vi "输入数据解析.vi"(0 "单个参数补充":dbl, 1 "从板号":dbl=1.0, 2 "主板二维码":string="BNET01", 3 "从板二维码":string="BNET01", 5 "主板引用":refnum<vi>, 7 "从板引用":refnum<vi>, 9 "主板选项":string="三级故障阀值", 11 "枚举":enum16{"主板", "从板"}(ring), 12 "快换":bool caption="快换写入") -> (4 "输出数组":dbl[][](array[numeric]), 6 "数组长度":dbl[](array[numeric]), 8 "循环次数":i32, 10 "命令":u32, 14 "名称":string[](array[string]), 15 "命令序号":u32[](array[numeric]))   [LabVIEW 2013] (continued)
                  disable-tunnel: [w3298 w3317] -> w3294
                  frame Disabled {
                    n1313 = Unbundle By Name(w3306) -> ("SOH过低"=w3305:dbl)
                    n1314 = call "输入分辨率计算-EV05.vi"("1字节?"=FALSE, "数值"=w3305, "偏移量"=0.0, "分辨率"=0.1) -> ("低字节"=w3307:dbl, "高字节1"=w3308:dbl)  [unwired: 1 in, 5 out]
                    n1315 = call "二进制解析-8.6.vi"("索引"=4, "数值"=w3308) -> ("低位子数组"=w3311:i32[])  [unwired: 3 out]
                    n1316 = call "二进制解析-8.6.vi"("索引"=4, "数值"=w3307) -> ("低位子数组"=w3300:i32[], "高位子数组"=w3310:i32[])  [unwired: 2 out]
                    n1317 = call "二进制解析-8.6.vi"("索引"=4, "数值"=0) -> ("低位子数组"=w3301:i32[])  [unwired: 3 out]
                    n1318 = Insert Into Array(array=w3311, new element=w3310) -> (w3304:i32[])  [unwired: 1 in]
                    n1319 = Insert Into Array(array=w3300, new element=w3301) -> (w3299:i32[])  [unwired: 1 in]
                    n1320 = call "数值二进制转十进制-8.6.vi"("子数组"=w3304) -> ("十进制数值"=w3309:i32)  [unwired: 4 out]
                    n1321 = call "数值二进制转十进制-8.6.vi"("子数组"=w3299) -> ("十进制数值"=w3298:i32)  [unwired: 4 out]
                  }
                  frame Enabled {
                    w3317 = 255 ("高字节1")
                  }
                }
                n1322 = Build Array(w3296, w3294) -> (w3297:i32[])
              }
            }
            n1323 = Insert Into Array(array=w3101, new element=w3102) -> (w3100:dbl[])  [unwired: 1 in]
          }
          n1324 = Build Array(w3097) -> (w3096:dbl[][])
          n1325 = Build Array("一级故障阀值") -> (w3087:string[])
        }
        frame "温度过低(2)" {
          n1326 = Unbundle By Name(w3323) -> ("一级故障 2"=w3324:refnum<vi>)
          n1327 = property class="Clust (严格)"(reference=w3324) -> ("Value"=w3322:T4)  [unwired: 1 in, 2 out]
          n1328 = for {
            N: 17 -> [_]
            tunnel: w3322 -> [w3334]
            shift-right: [w3331] -> w3328
            shift-left: dbl[] [] -> [w3332]
            i -> [w3335]
            n1329 = case shown="13" w3335 {
              tunnel: w3334 -> [w3336 w3347 w3358 w3368 w3378 w3388 w3400 w3412 w3424 w3436 w3448 w3460 w3474 w3496 w3508 w3517 w3526]
              tunnel: [w3337 w3348 w3359 w3369 w3379 w3390 w3402 w3414 w3426 w3438 w3450 w3461 w3483 w3499 w3507 w3516 w3528] -> w3333
              frame 0, Default {
                # "总电压过高"
                n1330 = disable-structure shown="启用" {
                  disable-tunnel: [w3343 w3346] -> w3339
                  disable-tunnel: [w3342 w3346] -> w3338
                  disable-tunnel: w3336 -> [w3341 _]
                  frame Disabled {
                    n1331 = Unbundle By Name(w3341) -> ("总电压过高"=w3340:dbl)
                    n1332 = call "输入分辨率计算-EV05.vi"("1字节?"=FALSE, "数值"=w3340, "分辨率"=0.1) -> ("低字节"=w3343:dbl, "高字节1"=w3342:dbl)  [unwired: 2 in, 5 out]
                  }
                  frame Enabled {
                    w3346 = 255 ("高字节1")
                  }
                }
                n1333 = Build Array(w3338, w3339) -> (w3337:i32[])
              }
              frame 1 {
                # "总电压过低"
                n1334 = disable-structure shown="启用" {
                  disable-tunnel: [w3354 w3357] -> w3350
                  disable-tunnel: [w3353 w3357] -> w3349
                  disable-tunnel: w3347 -> [w3352 _]
                  frame Disabled {
                    n1335 = Unbundle By Name(w3352) -> ("总电压过低"=w3351:dbl)
                    n1336 = call "输入分辨率计算-EV05.vi"("1字节?"=FALSE, "数值"=w3351, "分辨率"=0.1) -> ("低字节"=w3354:dbl, "高字节1"=w3353:dbl)  [unwired: 2 in, 5 out]
                  }
                  frame Enabled {
                    w3357 = 255 ("高字节1")
                  }
                }
                n1337 = Build Array(w3349, w3350) -> (w3348:i32[])
              }
              frame 2 {
                # "温度过高"
                n1338 = disable-structure shown="启用" {
                  disable-tunnel: [w3364 255 ("高字节1")] -> w3360
                  disable-tunnel: w3358 -> [w3362 _]
                  frame Disabled {
                    n1339 = Unbundle By Name(w3362) -> ("温度过高"=w3361:dbl)
                    n1340 = call "输入分辨率计算-EV05.vi"("1字节?"=TRUE, "数值"=w3361, "偏移量"=-40.0, "分辨率"=1.0) -> ("高字节1"=w3364:dbl)  [unwired: 1 in, 6 out]
                  }
                  frame Enabled {
                  }
                }
                n1341 = Build Array(w3360) -> (w3359:i32[])
              }
              frame 3 {
                # "温度过低"
                n1342 = disable-structure shown="启用" {
                  disable-tunnel: [w3374 255 ("高字节1")] -> w3370
                  disable-tunnel: w3368 -> [w3372 _]
                  frame Enabled {
                    n1343 = Unbundle By Name(w3372) -> ("温度过低"=w3371:dbl)
                    n1344 = call "输入分辨率计算-EV05.vi"("1字节?"=TRUE, "数值"=w3371, "偏移量"=-40.0, "分辨率"=1.0) -> ("高字节1"=w3374:dbl)  [unwired: 1 in, 6 out]
                  }
                  frame Disabled {
                  }
                }
                n1345 = Build Array(w3370) -> (w3369:dbl[])
              }
              frame 4 {
                # "整组温度不均衡"
                n1346 = disable-structure shown="启用" {
                  disable-tunnel: [w3384 255 ("高字节1")] -> w3380
                  disable-tunnel: w3378 -> [w3382 _]
                  frame Disabled {
                    n1347 = Unbundle By Name(w3382) -> ("整组温度不均衡"=w3381:dbl)
                    n1348 = call "输入分辨率计算-EV05.vi"("1字节?"=TRUE, "数值"=w3381, "偏移量"=0.0, "分辨率"=1.0) -> ("高字节1"=w3384:dbl)  [unwired: 1 in, 6 out]
                  }
                  frame Enabled {
                  }
                }
                n1349 = Build Array(w3380) -> (w3379:i32[])
              }
              frame 5 {
                # "单组电压不均衡"
                n1350 = disable-structure shown="启用" {
                  disable-tunnel: [w3396 w3399] -> w3391
                  disable-tunnel: [w3394 w3399] -> w3389
                  disable-tunnel: w3388 -> [w3393 _]
                  frame Disabled {
                    n1351 = Unbundle By Name(w3393) -> ("单组电压不均衡"=w3392:dbl)
                    n1352 = call "输入分辨率计算-EV05.vi"("1字节?"=FALSE, "数值"=w3392, "偏移量"=0.0, "分辨率"=0.001) -> ("低字节"=w3394:dbl, "高字节1"=w3396:dbl)  [unwired: 1 in, 5 out]
                  }
                  frame Enabled {
                    w3399 = 255 ("高字节1")
                  }
                }
                n1353 = Build Array(w3391, w3389) -> (w3390:i32[])
              }
              frame 6 {
                # "整组电压不均衡"
                n1354 = disable-structure shown="启用" {
                  disable-tunnel: [w3408 w3411] -> w3403
                  disable-tunnel: [w3406 w3411] -> w3401
                  disable-tunnel: w3400 -> [w3405 _]
                  frame Disabled {
                    n1355 = Unbundle By Name(w3405) -> ("整组电压不均衡"=w3404:dbl)
                    n1356 = call "输入分辨率计算-EV05.vi"("1字节?"=FALSE, "数值"=w3404, "偏移量"=0.0, "分辨率"=0.001) -> ("低字节"=w3406:dbl, "高字节1"=w3408:dbl)  [unwired: 1 in, 5 out]
                  }
                  frame Enabled {
                    w3411 = 255 ("高字节1")
                  }
                }
                n1357 = Build Array(w3403, w3401) -> (w3402:i32[])
              }
              frame 7 {
                # "单体电压过高"
                n1358 = disable-structure shown="启用" {
                  disable-tunnel: [w3420 w3423] -> w3415
                  disable-tunnel: [w3418 w3423] -> w3413
                  disable-tunnel: w3412 -> [w3417 _]
                  frame Disabled {
                    n1359 = Unbundle By Name(w3417) -> ("单体电压过高"=w3416:dbl)
                    n1360 = call "输入分辨率计算-EV05.vi"("1字节?"=FALSE, "数值"=w3416, "偏移量"=0.0, "分辨率"=0.001) -> ("低字节"=w3418:dbl, "高字节1"=w3420:dbl)  [unwired: 1 in, 5 out]
                  }
                  frame Enabled {
                    w3423 = 255 ("高字节1")
                  }
                }
                n1361 = Build Array(w3415, w3413) -> (w3414:i32[])
              }
              frame 8 {
                # "单体电压过低"
                n1362 = disable-structure shown="启用" {
                  disable-tunnel: [w3432 w3435] -> w3427
                  disable-tunnel: [w3430 w3435] -> w3425
                  disable-tunnel: w3424 -> [w3429 _]
                  frame Disabled {
                    n1363 = Unbundle By Name(w3429) -> ("单体电压过低"=w3428:dbl)
                    n1364 = call "输入分辨率计算-EV05.vi"("1字节?"=FALSE, "数值"=w3428, "偏移量"=0.0, "分辨率"=0.001) -> ("低字节"=w3430:dbl, "高字节1"=w3432:dbl)  [unwired: 1 in, 5 out]
                  }
                  frame Enabled {
                    w3435 = 255 ("高字节1")
                  }
                }
                n1365 = Build Array(w3427, w3425) -> (w3426:i32[])
              }
              frame 9 {
                # "充电电流过高"
                n1366 = disable-structure shown="启用" {
                  disable-tunnel: [w3444 w3447] -> w3439
                  disable-tunnel: [w3442 w3447] -> w3437
                  disable-tunnel: w3436 -> [w3441 _]
                  frame Disabled {
                    n1367 = Unbundle By Name(w3441) -> ("充电电流过高"=w3440:dbl)
                    n1368 = call "输入分辨率计算-EV05.vi"("1字节?"=FALSE, "数值"=w3440, "偏移量"=-3000.0, "分辨率"=0.1) -> ("低字节"=w3442:dbl, "高字节1"=w3444:dbl)  [unwired: 1 in, 5 out]
                  }
                  frame Enabled {
                    w3447 = 255 ("高字节1")
                  }
                }
                n1369 = Build Array(w3439, w3437) -> (w3438:i32[])
              }
              frame 10 {
                # "放电电流过高"
                n1370 = disable-structure shown="启用" {
                  disable-tunnel: [w3456 w3459] -> w3451
                  disable-tunnel: [w3454 w3459] -> w3449
                  disable-tunnel: w3448 -> [w3453 _]
                  frame Disabled {
                    n1371 = Unbundle By Name(w3453) -> ("放电电流过高"=w3452:dbl)
                    n1372 = call "输入分辨率计算-EV05.vi"("1字节?"=FALSE, "数值"=w3452, "偏移量"=-3000.0, "分辨率"=0.1) -> ("低字节"=w3454:dbl, "高字节1"=w3456:dbl)  [unwired: 1 in, 5 out]
                  }
                  frame Enabled {
                    w3459 = 255 ("高字节1")
                  }
                }
                n1373 = Build Array(w3451, w3449) -> (w3450:i32[])
              }
              frame 11 {
                # "单组温度不均衡"
                n1374 = disable-structure shown="启用" {
                  disable-tunnel: [w3466 255 ("高字节1")] -> w3462
                  disable-tunnel: w3460 -> [w3464 _]
                  frame Disabled {
                    n1375 = Unbundle By Name(w3464) -> ("单组温度不均衡"=w3463:dbl)
                    n1376 = call "输入分辨率计算-EV05.vi"("1字节?"=TRUE, "数值"=w3463, "偏移量"=0.0, "分辨率"=1.0) -> ("高字节1"=w3466:dbl)  [unwired: 1 in, 6 out]
                  }
                  frame Enabled {
                  }
                }
                n1377 = Build Array(w3462) -> (w3461:i32[])
              }
              frame 12 {
                # "SOC过高"
                n1378 = Unbundle By Name(w3474) -> ("SOC过高"=w3473:dbl)
                n1379 = call "输入分辨率计算-EV05.vi"("1字节?"=FALSE, "数值"=w3473, "偏移量"=0.0, "分辨率"=0.1) -> ("低字节"=w3475:dbl, "高字节1"=w3476:dbl)  [unwired: 1 in, 5 out]
                n1380 = call "二进制解析-8.6.vi"("索引"=4, "数值"=w3476) -> ("低位子数组"=w3479:i32[])  [unwired: 3 out]
                n1381 = call "二进制解析-8.6.vi"("索引"=4, "数值"=w3475) -> ("低位子数组"=w3471:i32[], "高位子数组"=w3478:i32[])  [unwired: 2 out]
                n1382 = Insert Into Array(array=w3479, new element=w3478) -> (w3477:i32[])  [unwired: 1 in]
                n1383 = call "数值二进制转十进制-8.6.vi"("子数组"=w3477) -> ("十进制数值"=w3472:i32)  [unwired: 4 out]
                n1384 = disable-structure shown="启用" {
                  disable-tunnel: w3472 -> [w3487 _]
                  disable-tunnel: [w3487 255 ("高字节1")] -> w3470
                  disable-tunnel: [w3486 i32[] [] ("低位子数组 21")] -> _
                  disable-tunnel: w3471 -> [w3486 _]
                  frame Disabled {
                  }
                  frame Enabled {
                  }
                }
                n1385 = Build Array(w3470, w3470) -> (w3483:i32[])
              }
              frame 13 {
                # "SOC过低"
                n1386 = Unbundle By Name(w3496) -> ("SOC过低"=w3495:dbl)
                n1387 = call "输入分辨率计算-EV05.vi"("1字节?"=FALSE, "数值"=w3495, "偏移量"=0.0, "分辨率"=0.1) -> ("低字节"=w3493:dbl, "高字节1"=w3494:dbl)  [unwired: 1 in, 5 out]
                n1388 = call "二进制解析-8.6.vi"("索引"=4, "数值"=w3494) -> ("低位子数组"=w3491:i32[])  [unwired: 3 out]
                n1389 = disable-structure shown="启用" {
                  disable-tunnel: w3493 -> [w3503 _]
                  disable-tunnel: [w3503 255 ("高字节1")] -> w3492
                  disable-tunnel: w3491 -> [w3502 _]
                  disable-tunnel: [_ 255 ("高字节1")] -> w3490
                  frame Disabled {
                    (unwired) i32[] [] ("低位子数组 4")
                  }
                  frame Enabled {
                  }
                }
                n1390 = Build Array(w3490, w3492) -> (w3499:i32[])
              }
              frame 14 {
                # "内阻过大"
                n1391 = disable-structure shown="启用" {
                  disable-tunnel: w3508 -> [w3513 _]
                  disable-tunnel: [w3509 255 ("高字节1")] -> w3506
                  frame Disabled {
                    n1392 = Unbundle By Name(w3513) -> ("内阻过大"=w3512:dbl)
                    n1393 = call "输入分辨率计算-EV05.vi"("1字节?"=TRUE, "数值"=w3512, "分辨率"=0.1) -> ("高字节1"=w3509:dbl)  [unwired: 2 in, 6 out]
                  }
                  frame Enabled {
                  }
                }
                n1394 = Build Array(w3506) -> (w3507:i32[])
              }
              frame 15 {
                # "极柱温度过高"
                n1395 = disable-structure shown="启用" {
                  disable-tunnel: w3517 -> [w3523 _]
                  disable-tunnel: [w3519 255 ("高字节1")] -> w3515
                  frame Disabled {
                    n1396 = Unbundle By Name(w3523) -> ("极柱温度过高"=w3522:dbl)
                    n1397 = call "输入分辨率计算-EV05.vi"("1字节?"=TRUE, "数值"=w3522, "偏移量"=-40.0, "分辨率"=1.0) -> ("高字节1"=w3519:dbl)  [unwired: 1 in, 6 out]
                  }
                  frame Enabled {
                  }
                }
                n1398 = Build Array(w3515) -> (w3516:i32[])
              }
              frame 16 {
                # "SOH过低"
                n1399 = disable-structure shown="启用" {
                  disable-tunnel: [w3540 w3548] -> w3527
                  disable-tunnel: w3526 -> [w3537 _]
                  disable-tunnel: [w3529 w3548] -> w3525
                  frame Disabled {
                    n1400 = Unbundle By Name(w3537) -> ("SOH过低"=w3536:dbl)
                    n1401 = call "输入分辨率计算-EV05.vi"("1字节?"=FALSE, "数值"=w3536, "偏移量"=0.0, "分辨率"=0.1) -> ("低字节"=w3538:dbl, "高字节1"=w3539:dbl)  [unwired: 1 in, 5 out]
                    n1402 = call "二进制解析-8.6.vi"("索引"=4, "数值"=w3539) -> ("低位子数组"=w3542:i32[])  [unwired: 3 out]
                    n1403 = call "二进制解析-8.6.vi"("索引"=4, "数值"=w3538) -> ("低位子数组"=w3531:i32[], "高位子数组"=w3541:i32[])  [unwired: 2 out]
                    n1404 = call "二进制解析-8.6.vi"("索引"=4, "数值"=0) -> ("低位子数组"=w3532:i32[])  [unwired: 3 out]
                    n1405 = Insert Into Array(array=w3542, new element=w3541) -> (w3535:i32[])  [unwired: 1 in]
                    n1406 = Insert Into Array(array=w3531, new element=w3532) -> (w3530:i32[])  [unwired: 1 in]
                    n1407 = call "数值二进制转十进制-8.6.vi"("子数组"=w3535) -> ("十进制数值"=w3540:i32)  [unwired: 4 out]
                    n1408 = call "数值二进制转十进制-8.6.vi"("子数组"=w3530) -> ("十进制数值"=w3529:i32)  [unwired: 4 out]
                  }
                  frame Enabled {
                    w3548 = 255 ("高字节1")
                  }
                }
                n1409 = Build Array(w3527, w3525) -> (w3528:i32[])
              }
            }
            n1410 = Insert Into Array(array=w3332, new element=w3333) -> (w3331:dbl[])  [unwired: 1 in]
          }
          n1411 = Build Array(w3328) -> (w3327:dbl[][])
          n1412 = Build Array("二级故障阀值") -> (w3318:string[])
        }
        frame "温度过低(3)" {
          n1413 = Unbundle By Name(w3554) -> ("一级故障 3"=w3555:refnum<vi>)
          n1414 = property class="Clust (严格)"(reference=w3555) -> ("Value"=w3553:T4)  [unwired: 1 in, 2 out]
          n1415 = for {
            N: 17 -> [_]
            tunnel: w3553 -> [w3565]
            shift-right: [w3562] -> w3559
            shift-left: dbl[] [] -> [w3563]
            i -> [w3566]
            n1416 = case shown="13" w3566 {
              tunnel: w3565 -> [w3567 w3578 w3589 w3599 w3609 w3619 w3631 w3643 w3655 w3667 w3679 w3691 w3705 w3727 w3739 w3748 w3757]
              tunnel: [w3568 w3579 w3590 w3600 w3610 w3621 w3633 w3645 w3657 w3669 w3681 w3692 w3714 w3730 w3738 w3747 w3759] -> w3564
              frame 0, Default {
                # "总电压过高"
                n1417 = disable-structure shown="启用" {
                  disable-tunnel: [w3574 w3577] -> w3570
                  disable-tunnel: [w3573 w3577] -> w3569
                  disable-tunnel: w3567 -> [w3572 _]
                  frame Disabled {
                    n1418 = Unbundle By Name(w3572) -> ("总电压过高"=w3571:dbl)
                    n1419 = call "输入分辨率计算-EV05.vi"("1字节?"=FALSE, "数值"=w3571, "分辨率"=0.1) -> ("低字节"=w3574:dbl, "高字节1"=w3573:dbl)  [unwired: 2 in, 5 out]
                  }
                  frame Enabled {
                    w3577 = 255 ("高字节1")
                  }
                }
                n1420 = Build Array(w3569, w3570) -> (w3568:i32[])
              }
              frame 1 {
                # "总电压过低"
                n1421 = disable-structure shown="启用" {
                  disable-tunnel: [w3585 w3588] -> w3581
                  disable-tunnel: [w3584 w3588] -> w3580
                  disable-tunnel: w3578 -> [w3583 _]
                  frame Disabled {
                    n1422 = Unbundle By Name(w3583) -> ("总电压过低"=w3582:dbl)
                    n1423 = call "输入分辨率计算-EV05.vi"("1字节?"=FALSE, "数值"=w3582, "分辨率"=0.1) -> ("低字节"=w3585:dbl, "高字节1"=w3584:dbl)  [unwired: 2 in, 5 out]
                  }
                  frame Enabled {
                    w3588 = 255 ("高字节1")
                  }
                }
                n1424 = Build Array(w3580, w3581) -> (w3579:i32[])
              }
              frame 2 {
                # "温度过高"
                n1425 = disable-structure shown="启用" {
                  disable-tunnel: [w3595 255 ("高字节1")] -> w3591
                  disable-tunnel: w3589 -> [w3593 _]
                  frame Disabled {
                    n1426 = Unbundle By Name(w3593) -> ("温度过高"=w3592:dbl)
                    n1427 = call "输入分辨率计算-EV05.vi"("1字节?"=TRUE, "数值"=w3592, "偏移量"=-40.0, "分辨率"=1.0) -> ("高字节1"=w3595:dbl)  [unwired: 1 in, 6 out]
                  }
                  frame Enabled {
                  }
                }
                n1428 = Build Array(w3591) -> (w3590:i32[])
              }
              frame 3 {
                # "温度过低"
                n1429 = disable-structure shown="启用" {
                  disable-tunnel: [w3605 255 ("高字节1")] -> w3601
                  disable-tunnel: w3599 -> [w3603 _]
                  frame Enabled {
                    n1430 = Unbundle By Name(w3603) -> ("温度过低"=w3602:dbl)
                    n1431 = call "输入分辨率计算-EV05.vi"("1字节?"=TRUE, "数值"=w3602, "偏移量"=-40.0, "分辨率"=1.0) -> ("高字节1"=w3605:dbl)  [unwired: 1 in, 6 out]
                  }
                  frame Disabled {
                  }
                }
                n1432 = Build Array(w3601) -> (w3600:dbl[])
              }
              frame 4 {
                # "整组温度不均衡"
                n1433 = disable-structure shown="启用" {
                  disable-tunnel: [w3615 255 ("高字节1")] -> w3611
                  disable-tunnel: w3609 -> [w3613 _]
                  frame Disabled {
                    n1434 = Unbundle By Name(w3613) -> ("整组温度不均衡"=w3612:dbl)
                    n1435 = call "输入分辨率计算-EV05.vi"("1字节?"=TRUE, "数值"=w3612, "偏移量"=0.0, "分辨率"=1.0) -> ("高字节1"=w3615:dbl)  [unwired: 1 in, 6 out]
                  }
                  frame Enabled {
                  }
                }
                n1436 = Build Array(w3611) -> (w3610:i32[])
              }
              frame 5 {
                # "单组电压不均衡"
                n1437 = disable-structure shown="启用" {
                  disable-tunnel: [w3627 w3630] -> w3622
                  disable-tunnel: [w3625 w3630] -> w3620
                  disable-tunnel: w3619 -> [w3624 _]
                  frame Disabled {
                    n1438 = Unbundle By Name(w3624) -> ("单组电压不均衡"=w3623:dbl)
                    n1439 = call "输入分辨率计算-EV05.vi"("1字节?"=FALSE, "数值"=w3623, "偏移量"=0.0, "分辨率"=0.001) -> ("低字节"=w3625:dbl, "高字节1"=w3627:dbl)  [unwired: 1 in, 5 out]
                  }
                  frame Enabled {
                    w3630 = 255 ("高字节1")
                  }
                }
                n1440 = Build Array(w3622, w3620) -> (w3621:i32[])
              }
              frame 6 {
                # "整组电压不均衡"
                n1441 = disable-structure shown="启用" {
                  disable-tunnel: [w3639 w3642] -> w3634
                  disable-tunnel: [w3637 w3642] -> w3632
                  disable-tunnel: w3631 -> [w3636 _]
                  frame Disabled {
                    n1442 = Unbundle By Name(w3636) -> ("整组电压不均衡"=w3635:dbl)
                    n1443 = call "输入分辨率计算-EV05.vi"("1字节?"=FALSE, "数值"=w3635, "偏移量"=0.0, "分辨率"=0.001) -> ("低字节"=w3637:dbl, "高字节1"=w3639:dbl)  [unwired: 1 in, 5 out]
                  }
                  frame Enabled {
                    w3642 = 255 ("高字节1")
                  }
                }
                n1444 = Build Array(w3634, w3632) -> (w3633:i32[])
              }
              frame 7 {
                # "单体电压过高"
                n1445 = disable-structure shown="启用" {
                  disable-tunnel: [w3651 w3654] -> w3646
                  disable-tunnel: [w3649 w3654] -> w3644
                  disable-tunnel: w3643 -> [w3648 _]
                  frame Disabled {
                    n1446 = Unbundle By Name(w3648) -> ("单体电压过高"=w3647:dbl)
                    n1447 = call "输入分辨率计算-EV05.vi"("1字节?"=FALSE, "数值"=w3647, "偏移量"=0.0, "分辨率"=0.001) -> ("低字节"=w3649:dbl, "高字节1"=w3651:dbl)  [unwired: 1 in, 5 out]
                  }
                  frame Enabled {
                    w3654 = 255 ("高字节1")
                  }
                }
                n1448 = Build Array(w3646, w3644) -> (w3645:i32[])
              }
              frame 8 {
                # "单体电压过低"
                n1449 = disable-structure shown="启用" {
                  disable-tunnel: [w3663 w3666] -> w3658
                  disable-tunnel: [w3661 w3666] -> w3656
                  disable-tunnel: w3655 -> [w3660 _]
                  frame Disabled {
                    n1450 = Unbundle By Name(w3660) -> ("单体电压过低"=w3659:dbl)
                    n1451 = call "输入分辨率计算-EV05.vi"("1字节?"=FALSE, "数值"=w3659, "偏移量"=0.0, "分辨率"=0.001) -> ("低字节"=w3661:dbl, "高字节1"=w3663:dbl)  [unwired: 1 in, 5 out]
                  }
                  frame Enabled {
                    w3666 = 255 ("高字节1")
                  }
                }
                n1452 = Build Array(w3658, w3656) -> (w3657:i32[])
              }
              frame 9 {
                # "充电电流过高"
                n1453 = disable-structure shown="启用" {
                  disable-tunnel: [w3675 w3678] -> w3670
                  disable-tunnel: [w3673 w3678] -> w3668
                  disable-tunnel: w3667 -> [w3672 _]
                  frame Disabled {
                    n1454 = Unbundle By Name(w3672) -> ("充电电流过高"=w3671:dbl)
                    n1455 = call "输入分辨率计算-EV05.vi"("1字节?"=FALSE, "数值"=w3671, "偏移量"=-3000.0, "分辨率"=0.1) -> ("低字节"=w3673:dbl, "高字节1"=w3675:dbl)  [unwired: 1 in, 5 out]
                  }
                  frame Enabled {
                    w3678 = 255 ("高字节1")
                  }
                }
                n1456 = Build Array(w3670, w3668) -> (w3669:i32[])
              }
              frame 10 {
                # "放电电流过高"
                n1457 = disable-structure shown="启用" {
                  disable-tunnel: [w3687 w3690] -> w3682
                  disable-tunnel: [w3685 w3690] -> w3680
                  disable-tunnel: w3679 -> [w3684 _]
                  frame Disabled {
                    n1458 = Unbundle By Name(w3684) -> ("放电电流过高"=w3683:dbl)
                    n1459 = call "输入分辨率计算-EV05.vi"("1字节?"=FALSE, "数值"=w3683, "偏移量"=-3000.0, "分辨率"=0.1) -> ("低字节"=w3685:dbl, "高字节1"=w3687:dbl)  [unwired: 1 in, 5 out]
                  }
                  frame Enabled {
                    w3690 = 255 ("高字节1")
                  }
                }
                n1460 = Build Array(w3682, w3680) -> (w3681:i32[])
              }
              frame 11 {
                # "单组温度不均衡"
                n1461 = disable-structure shown="启用" {
                  disable-tunnel: [w3697 255 ("高字节1")] -> w3693
                  disable-tunnel: w3691 -> [w3695 _]
                  frame Disabled {
                    n1462 = Unbundle By Name(w3695) -> ("单组温度不均衡"=w3694:dbl)
                    n1463 = call "输入分辨率计算-EV05.vi"("1字节?"=TRUE, "数值"=w3694, "偏移量"=0.0, "分辨率"=1.0) -> ("高字节1"=w3697:dbl)  [unwired: 1 in, 6 out]
                  }
                  frame Enabled {
                  }
                }
                n1464 = Build Array(w3693) -> (w3692:i32[])
              }
              frame 12 {
                # "SOC过高"
                n1465 = Unbundle By Name(w3705) -> ("SOC过高"=w3704:dbl)
                n1466 = call "输入分辨率计算-EV05.vi"("1字节?"=FALSE, "数值"=w3704, "偏移量"=0.0, "分辨率"=0.1) -> ("低字节"=w3706:dbl, "高字节1"=w3707:dbl)  [unwired: 1 in, 5 out]
                n1467 = call "二进制解析-8.6.vi"("索引"=4, "数值"=w3707) -> ("低位子数组"=w3710:i32[])  [unwired: 3 out]
                n1468 = call "二进制解析-8.6.vi"("索引"=4, "数值"=w3706) -> ("低位子数组"=w3702:i32[], "高位子数组"=w3709:i32[])  [unwired: 2 out]
                n1469 = Insert Into Array(array=w3710, new element=w3709) -> (w3708:i32[])  [unwired: 1 in]
                n1470 = call "数值二进制转十进制-8.6.vi"("子数组"=w3708) -> ("十进制数值"=w3703:i32)  [unwired: 4 out]
                n1471 = disable-structure shown="启用" {
                  disable-tunnel: w3703 -> [w3718 _]
                  disable-tunnel: [w3718 255 ("高字节1")] -> w3701
                  disable-tunnel: [w3717 i32[] [] ("低位子数组 21")] -> _
                  disable-tunnel: w3702 -> [w3717 _]
                  frame Disabled {
                  }
                  frame Enabled {
                  }
                }
                n1472 = Build Array(w3701, w3701) -> (w3714:i32[])
              }
              frame 13 {
                # "SOC过低"
                n1473 = Unbundle By Name(w3727) -> ("SOC过低"=w3726:dbl)
                n1474 = call "输入分辨率计算-EV05.vi"("1字节?"=FALSE, "数值"=w3726, "偏移量"=0.0, "分辨率"=0.1) -> ("低字节"=w3724:dbl, "高字节1"=w3725:dbl)  [unwired: 1 in, 5 out]
                n1475 = call "二进制解析-8.6.vi"("索引"=4, "数值"=w3725) -> ("低位子数组"=w3722:i32[])  [unwired: 3 out]
                n1476 = disable-structure shown="启用" {
                  disable-tunnel: w3724 -> [w3734 _]
                  disable-tunnel: [w3734 255 ("高字节1")] -> w3723
                  disable-tunnel: w3722 -> [w3733 _]
                  disable-tunnel: [_ 255 ("高字节1")] -> w3721
                  frame Disabled {
                    (unwired) i32[] [] ("低位子数组 4")
                  }
                  frame Enabled {
                  }
                }
                n1477 = Build Array(w3721, w3723) -> (w3730:i32[])
              }
              frame 14 {
                # "内阻过大"
                n1478 = disable-structure shown="启用" {
                  disable-tunnel: w3739 -> [w3744 _]
                  disable-tunnel: [w3740 255 ("高字节1")] -> w3737
                  frame Disabled {
                    n1479 = Unbundle By Name(w3744) -> ("内阻过大"=w3743:dbl)
                    n1480 = call "输入分辨率计算-EV05.vi"("1字节?"=TRUE, "数值"=w3743, "分辨率"=0.1) -> ("高字节1"=w3740:dbl)  [unwired: 2 in, 6 out]
                  }
                  frame Enabled {
                  }
                }
                n1481 = Build Array(w3737) -> (w3738:i32[])
              }
              frame 15 {
                # "极柱温度过高"
                n1482 = disable-structure shown="启用" {
                  disable-tunnel: w3748 -> [w3754 _]
                  disable-tunnel: [w3750 255 ("高字节1")] -> w3746
                  frame Disabled {
                    n1483 = Unbundle By Name(w3754) -> ("极柱温度过高"=w3753:dbl)
                    n1484 = call "输入分辨率计算-EV05.vi"("1字节?"=TRUE, "数值"=w3753, "偏移量"=-40.0, "分辨率"=1.0) -> ("高字节1"=w3750:dbl)  [unwired: 1 in, 6 out]
                  }
                  frame Enabled {
                  }
                }
                n1485 = Build Array(w3746) -> (w3747:i32[])
              }
              frame 16 {
                # "SOH过低"
                n1486 = disable-structure shown="启用" {
                  disable-tunnel: [w3771 w3779] -> w3758
                  disable-tunnel: w3757 -> [w3768 _]
                  disable-tunnel: [w3760 w3779] -> w3756
                  frame Disabled {
                    n1487 = Unbundle By Name(w3768) -> ("SOH过低"=w3767:dbl)
                    n1488 = call "输入分辨率计算-EV05.vi"("1字节?"=FALSE, "数值"=w3767, "偏移量"=0.0, "分辨率"=0.1) -> ("低字节"=w3769:dbl, "高字节1"=w3770:dbl)  [unwired: 1 in, 5 out]
                    n1489 = call "二进制解析-8.6.vi"("索引"=4, "数值"=w3770) -> ("低位子数组"=w3773:i32[])  [unwired: 3 out]
                    n1490 = call "二进制解析-8.6.vi"("索引"=4, "数值"=w3769) -> ("低位子数组"=w3762:i32[], "高位子数组"=w3772:i32[])  [unwired: 2 out]
                    n1491 = call "二进制解析-8.6.vi"("索引"=4, "数值"=0) -> ("低位子数组"=w3763:i32[])  [unwired: 3 out]
                    n1492 = Insert Into Array(array=w3773, new element=w3772) -> (w3766:i32[])  [unwired: 1 in]
                    n1493 = Insert Into Array(array=w3762, new element=w3763) -> (w3761:i32[])  [unwired: 1 in]
                    n1494 = call "数值二进制转十进制-8.6.vi"("子数组"=w3766) -> ("十进制数值"=w3771:i32)  [unwired: 4 out]
                    n1495 = call "数值二进制转十进制-8.6.vi"("子数组"=w3761) -> ("十进制数值"=w3760:i32)  [unwired: 4 out]
                  }
                  frame Enabled {
                    w3779 = 255 ("高字节1")
                  }
                }
                n1496 = Build Array(w3758, w3756) -> (w3759:i32[])
              }
            }
            n1497 = Insert Into Array(array=w3563, new element=w3564) -> (w3562:dbl[])  [unwired: 1 in]
          }
          n1498 = Build Array(w3559) -> (w3558:dbl[][])
          n1499 = Build Array("三级故障阀值") -> (w3549:string[])
        }
        frame "整组温度不均衡" {
          n1500 = Unbundle By Name(w3785) -> ("一级故障"=w3786:refnum<vi>)
          n1501 = property class="Clust (严格)"(reference=w3786) -> ("Value"=w3784:T4)  [unwired: 1 in, 2 out]
          n1502 = for {
            N: 17 -> [_]
            tunnel: w3784 -> [w3796]
            shift-right: [w3793] -> w3790
            shift-left: dbl[] [] -> [w3794]
            i -> [w3797]
            n1503 = case shown="11" w3797 {
              tunnel: w3796 -> [w3798 w3809 w3820 w3830 w3840 w3849 w3861 w3873 w3885 w3897 w3909 w3921 w3935 w3957 w3969 w3978 w3987]
              tunnel: [w3799 w3810 w3821 w3831 w3841 w3851 w3863 w3875 w3887 w3899 w3911 w3922 w3944 w3960 w3968 w3977 w3989] -> w3795
              frame 0, Default {
                # "总电压过高"
                n1504 = disable-structure shown="启用" {
                  disable-tunnel: [w3805 w3808] -> w3801
                  disable-tunnel: [w3804 w3808] -> w3800
                  disable-tunnel: w3798 -> [w3803 _]
                  frame Disabled {
                    n1505 = Unbundle By Name(w3803) -> ("总电压过高"=w3802:dbl)
                    n1506 = call "输入分辨率计算-EV05.vi"("1字节?"=FALSE, "数值"=w3802, "分辨率"=0.1) -> ("低字节"=w3805:dbl, "高字节1"=w3804:dbl)  [unwired: 2 in, 5 out]
                  }
                  frame Enabled {
                    w3808 = 255 ("高字节1")
                  }
                }
                n1507 = Build Array(w3800, w3801) -> (w3799:i32[])
              }
              frame 1 {
                # "总电压过低"
                n1508 = disable-structure shown="启用" {
                  disable-tunnel: [w3816 w3819] -> w3812
                  disable-tunnel: [w3815 w3819] -> w3811
                  disable-tunnel: w3809 -> [w3814 _]
                  frame Disabled {
                    n1509 = Unbundle By Name(w3814) -> ("总电压过低"=w3813:dbl)
                    n1510 = call "输入分辨率计算-EV05.vi"("1字节?"=FALSE, "数值"=w3813, "分辨率"=0.1) -> ("低字节"=w3816:dbl, "高字节1"=w3815:dbl)  [unwired: 2 in, 5 out]
                  }
                  frame Enabled {
                    w3819 = 255 ("高字节1")
                  }
                }
                n1511 = Build Array(w3811, w3812) -> (w3810:i32[])
              }
              frame 2 {
                # "温度过高"
                n1512 = disable-structure shown="启用" {
                  disable-tunnel: [w3826 255 ("高字节1")] -> w3822
                  disable-tunnel: w3820 -> [w3824 _]
                  frame Disabled {
                    n1513 = Unbundle By Name(w3824) -> ("温度过高"=w3823:dbl)
                    n1514 = call "输入分辨率计算-EV05.vi"("1字节?"=TRUE, "数值"=w3823, "偏移量"=-40.0, "分辨率"=1.0) -> ("高字节1"=w3826:dbl)  [unwired: 1 in, 6 out]
                  }
                  frame Enabled {
                  }
                }
                n1515 = Build Array(w3822) -> (w3821:i32[])
              }
              frame 3 {
                # "温度过低"
                n1516 = disable-structure shown="启用" {
                  disable-tunnel: [w3836 255 ("高字节1")] -> w3832
                  disable-tunnel: w3830 -> [w3834 _]
                  frame Disabled {
                    n1517 = Unbundle By Name(w3834) -> ("温度过低"=w3833:dbl)
                    n1518 = call "输入分辨率计算-EV05.vi"("1字节?"=TRUE, "数值"=w3833, "偏移量"=-40.0, "分辨率"=1.0) -> ("高字节1"=w3836:dbl)  [unwired: 1 in, 6 out]
                  }
                  frame Enabled {
                  }
                }
                n1519 = Build Array(w3832) -> (w3831:i32[])
              }
              frame 4 {
                # "整组温度不均衡"
                n1520 = disable-structure shown="启用" {
                  disable-tunnel: [w3845 255 ("高字节1")] -> w3842
                  disable-tunnel: w3840 -> [w3844 _]
                  frame Enabled {
                    n1521 = Unbundle By Name(w3844) -> ("整组温度不均衡"=w3843:dbl)
                    n1522 = call "输入分辨率计算-EV05.vi"("1字节?"=TRUE, "数值"=w3843, "分辨率"=1.0) -> ("高字节1"=w3845:dbl)  [unwired: 2 in, 6 out]
                  }
                  frame Disabled {
                  }
                }
                n1523 = Build Array(w3842) -> (w3841:dbl[])
              }
              frame 5 {
                # "单组电压不均衡"
                n1524 = disable-structure shown="启用" {
                  disable-tunnel: [w3857 w3860] -> w3852
                  disable-tunnel: [w3855 w3860] -> w3850
                  disable-tunnel: w3849 -> [w3854 _]
                  frame Disabled {
                    n1525 = Unbundle By Name(w3854) -> ("单组电压不均衡"=w3853:dbl)
                    n1526 = call "输入分辨率计算-EV05.vi"("1字节?"=FALSE, "数值"=w3853, "偏移量"=0.0, "分辨率"=0.001) -> ("低字节"=w3855:dbl, "高字节1"=w3857:dbl)  [unwired: 1 in, 5 out]
                  }
                  frame Enabled {
                    w3860 = 255 ("高字节1")
                  }
                }
                n1527 = Build Array(w3852, w3850) -> (w3851:i32[])
              }
              frame 6 {
                # "整组电压不均衡"
                n1528 = disable-structure shown="启用" {
                  disable-tunnel: [w3869 w3872] -> w3864
                  disable-tunnel: [w3867 w3872] -> w3862
                  disable-tunnel: w3861 -> [w3866 _]
                  frame Disabled {
                    n1529 = Unbundle By Name(w3866) -> ("整组电压不均衡"=w3865:dbl)
                    n1530 = call "输入分辨率计算-EV05.vi"("1字节?"=FALSE, "数值"=w3865, "偏移量"=0.0, "分辨率"=0.001) -> ("低字节"=w3867:dbl, "高字节1"=w3869:dbl)  [unwired: 1 in, 5 out]
                  }
                  frame Enabled {
                    w3872 = 255 ("高字节1")
                  }
                }
                n1531 = Build Array(w3864, w3862) -> (w3863:i32[])
              }
              frame 7 {
                # "单体电压过高"
                n1532 = disable-structure shown="启用" {
                  disable-tunnel: [w3881 w3884] -> w3876
                  disable-tunnel: [w3879 w3884] -> w3874
                  disable-tunnel: w3873 -> [w3878 _]
                  frame Disabled {
                    n1533 = Unbundle By Name(w3878) -> ("单体电压过高"=w3877:dbl)
                    n1534 = call "输入分辨率计算-EV05.vi"("1字节?"=FALSE, "数值"=w3877, "偏移量"=0.0, "分辨率"=0.001) -> ("低字节"=w3879:dbl, "高字节1"=w3881:dbl)  [unwired: 1 in, 5 out]
                  }
                  frame Enabled {
                    w3884 = 255 ("高字节1")
                  }
                }
                n1535 = Build Array(w3876, w3874) -> (w3875:i32[])
              }
              frame 8 {
                # "单体电压过低"
                n1536 = disable-structure shown="启用" {
                  disable-tunnel: [w3893 w3896] -> w3888
                  disable-tunnel: [w3891 w3896] -> w3886
                  disable-tunnel: w3885 -> [w3890 _]
                  frame Disabled {
                    n1537 = Unbundle By Name(w3890) -> ("单体电压过低"=w3889:dbl)
                    n1538 = call "输入分辨率计算-EV05.vi"("1字节?"=FALSE, "数值"=w3889, "偏移量"=0.0, "分辨率"=0.001) -> ("低字节"=w3891:dbl, "高字节1"=w3893:dbl)  [unwired: 1 in, 5 out]
                  }
                  frame Enabled {
                    w3896 = 255 ("高字节1")
                  }
                }
                n1539 = Build Array(w3888, w3886) -> (w3887:i32[])
              }
              frame 9 {
                # "充电电流过高"
                n1540 = disable-structure shown="启用" {
                  disable-tunnel: [w3905 w3908] -> w3900
                  disable-tunnel: [w3903 w3908] -> w3898
                  disable-tunnel: w3897 -> [w3902 _]
                  frame Disabled {
                    n1541 = Unbundle By Name(w3902) -> ("充电电流过高"=w3901:dbl)
                    n1542 = call "输入分辨率计算-EV05.vi"("1字节?"=FALSE, "数值"=w3901, "偏移量"=-3000.0, "分辨率"=0.1) -> ("低字节"=w3903:dbl, "高字节1"=w3905:dbl)  [unwired: 1 in, 5 out]
                  }
                  frame Enabled {
                    w3908 = 255 ("高字节1")
                  }
                }
                n1543 = Build Array(w3900, w3898) -> (w3899:i32[])
              }
              frame 10 {
                # "放电电流过高"
                n1544 = disable-structure shown="启用" {
                  disable-tunnel: [w3917 w3920] -> w3912
                  disable-tunnel: [w3915 w3920] -> w3910
                  disable-tunnel: w3909 -> [w3914 _]
                  frame Disabled {
                    n1545 = Unbundle By Name(w3914) -> ("放电电流过高"=w3913:dbl)
                    n1546 = call "输入分辨率计算-EV05.vi"("1字节?"=FALSE, "数值"=w3913, "偏移量"=-3000.0, "分辨率"=0.1) -> ("低字节"=w3915:dbl, "高字节1"=w3917:dbl)  [unwired: 1 in, 5 out]
                  }
                  frame Enabled {
                    w3920 = 255 ("高字节1")
                  }
                }
                n1547 = Build Array(w3912, w3910) -> (w3911:i32[])
              }
              frame 11 {
                # "单组温度不均衡"
                n1548 = disable-structure shown="启用" {
                  disable-tunnel: [w3927 255 ("高字节1")] -> w3923
                  disable-tunnel: w3921 -> [w3925 _]
                  frame Disabled {
                    n1549 = Unbundle By Name(w3925) -> ("单组温度不均衡"=w3924:dbl)
                    n1550 = call "输入分辨率计算-EV05.vi"("1字节?"=TRUE, "数值"=w3924, "偏移量"=0.0, "分辨率"=1.0) -> ("高字节1"=w3927:dbl)  [unwired: 1 in, 6 out]
                  }
                  frame Enabled {
                  }
                }
                n1551 = Build Array(w3923) -> (w3922:i32[])
              }
              frame 12 {
                # "SOC过高"
                n1552 = Unbundle By Name(w3935) -> ("SOC过高"=w3934:dbl)
                n1553 = call "输入分辨率计算-EV05.vi"("1字节?"=FALSE, "数值"=w3934, "偏移量"=0.0, "分辨率"=0.1) -> ("低字节"=w3936:dbl, "高字节1"=w3937:dbl)  [unwired: 1 in, 5 out]
                n1554 = call "二进制解析-8.6.vi"("索引"=4, "数值"=w3937) -> ("低位子数组"=w3940:i32[])  [unwired: 3 out]
                n1555 = call "二进制解析-8.6.vi"("索引"=4, "数值"=w3936) -> ("低位子数组"=w3932:i32[], "高位子数组"=w3939:i32[])  [unwired: 2 out]
                n1556 = Insert Into Array(array=w3940, new element=w3939) -> (w3938:i32[])  [unwired: 1 in]
                n1557 = call "数值二进制转十进制-8.6.vi"("子数组"=w3938) -> ("十进制数值"=w3933:i32)  [unwired: 4 out]
                n1558 = disable-structure shown="禁用" {
                  disable-tunnel: w3933 -> [w3948 _]
                  disable-tunnel: [w3948 255 ("高字节1")] -> w3931
                  disable-tunnel: [w3947 i32[] [] ("低位子数组 22")] -> _
                  disable-tunnel: w3932 -> [w3947 _]
                  frame Disabled {
                  }
                  frame Enabled {
                  }
                }
                n1559 = Build Array(w3931, w3931) -> (w3944:i32[])
              }
              frame 13 {
                # "SOC过低"
                n1560 = Unbundle By Name(w3957) -> ("SOC过低"=w3956:dbl)
                n1561 = call "输入分辨率计算-EV05.vi"("1字节?"=FALSE, "数值"=w3956, "偏移量"=0.0, "分辨率"=0.1) -> ("低字节"=w3954:dbl, "高字节1"=w3955:dbl)  [unwired: 1 in, 5 out]
                n1562 = call "二进制解析-8.6.vi"("索引"=4, "数值"=w3955) -> ("低位子数组"=w3952:i32[])  [unwired: 3 out]
                n1563 = disable-structure shown="启用" {
                  disable-tunnel: w3954 -> [w3964 _]
                  disable-tunnel: [w3964 255 ("高字节1")] -> w3953
                  disable-tunnel: w3952 -> [w3963 _]
                  disable-tunnel: [_ 255 ("高字节1")] -> w3951
                  frame Disabled {
                    (unwired) i32[] [] ("低位子数组 4")
                  }
                  frame Enabled {
                  }
                }
                n1564 = Build Array(w3951, w3953) -> (w3960:i32[])
              }
              frame 14 {
                # "内阻过大"
                n1565 = disable-structure shown="启用" {
                  disable-tunnel: w3969 -> [w3974 _]
                  disable-tunnel: [w3970 255 ("高字节1")] -> w3967
                  frame Disabled {
                    n1566 = Unbundle By Name(w3974) -> ("内阻过大"=w3973:dbl)
                    n1567 = call "输入分辨率计算-EV05.vi"("1字节?"=TRUE, "数值"=w3973, "分辨率"=0.1) -> ("高字节1"=w3970:dbl)  [unwired: 2 in, 6 out]
                  }
                  frame Enabled {
                  }
                }
                n1568 = Build Array(w3967) -> (w3968:i32[])
              }
              frame 15 {
                # "极柱温度过高"
                n1569 = disable-structure shown="启用" {
                  disable-tunnel: w3978 -> [w3984 _]
                  disable-tunnel: [w3980 255 ("高字节1")] -> w3976
                  frame Disabled {
                    n1570 = Unbundle By Name(w3984) -> ("极柱温度过高"=w3983:dbl)
                    n1571 = call "输入分辨率计算-EV05.vi"("1字节?"=TRUE, "数值"=w3983, "偏移量"=-40.0, "分辨率"=1.0) -> ("高字节1"=w3980:dbl)  [unwired: 1 in, 6 out]
                  }
                  frame Enabled {
                  }
                }
                n1572 = Build Array(w3976) -> (w3977:i32[])
              }
              frame 16 {
                # "SOH过低"
                n1573 = disable-structure shown="启用" {
                  disable-tunnel: [w4001 w4009] -> w3988
                  disable-tunnel: w3987 -> [w3998 _]
                  disable-tunnel: [w3990 w4009] -> w3986
                  frame Disabled {
                    n1574 = Unbundle By Name(w3998) -> ("SOH过低"=w3997:dbl)
                    n1575 = call "输入分辨率计算-EV05.vi"("1字节?"=FALSE, "数值"=w3997, "偏移量"=0.0, "分辨率"=0.1) -> ("低字节"=w3999:dbl, "高字节1"=w4000:dbl)  [unwired: 1 in, 5 out]
                    n1576 = call "二进制解析-8.6.vi"("索引"=4, "数值"=w4000) -> ("低位子数组"=w4003:i32[])  [unwired: 3 out]
                    n1577 = call "二进制解析-8.6.vi"("索引"=4, "数值"=w3999) -> ("低位子数组"=w3992:i32[], "高位子数组"=w4002:i32[])  [unwired: 2 out]
                    n1578 = call "二进制解析-8.6.vi"("索引"=4, "数值"=0) -> ("低位子数组"=w3993:i32[])  [unwired: 3 out]
                    n1579 = Insert Into Array(array=w4003, new element=w4002) -> (w3996:i32[])  [unwired: 1 in]
                    n1580 = Insert Into Array(array=w3992, new element=w3993) -> (w3991:i32[])  [unwired: 1 in]
                    n1581 = call "数值二进制转十进制-8.6.vi"("子数组"=w3996) -> ("十进制数值"=w4001:i32)  [unwired: 4 out]
                    n1582 = call "数值二进制转十进制-8.6.vi"("子数组"=w3991) -> ("十进制数值"=w3990:i32)  [unwired: 4 out]
                  }
                  frame Enabled {
                    w4009 = 255 ("高字节1")
                  }
                }
                n1583 = Build Array(w3988, w3986) -> (w3989:i32[])
              }
            }
            n1584 = Insert Into Array(array=w3794, new element=w3795) -> (w3793:dbl[])  [unwired: 1 in]
          }
          n1585 = Build Array(w3790) -> (w3789:dbl[][])
          n1586 = Build Array("一级故障阀值") -> (w3780:string[])
        }
        frame "整组温度不均衡(2)" {
          n1587 = Unbundle By Name(w4015) -> ("一级故障 2"=w4016:refnum<vi>)
          n1588 = property class="Clust (严格)"(reference=w4016) -> ("Value"=w4014:T4)  [unwired: 1 in, 2 out]
          n1589 = for {
            N: 17 -> [_]
            tunnel: w4014 -> [w4026]
            shift-right: [w4023] -> w4020
            shift-left: dbl[] [] -> [w4024]
            i -> [w4027]
            n1590 = case shown="11" w4027 {
              tunnel: w4026 -> [w4028 w4039 w4050 w4060 w4070 w4079 w4091 w4103 w4115 w4127 w4139 w4151 w4165 w4187 w4199 w4208 w4217]
              tunnel: [w4029 w4040 w4051 w4061 w4071 w4081 w4093 w4105 w4117 w4129 w4141 w4152 w4174 w4190 w4198 w4207 w4219] -> w4025
              frame 0, Default {
                # "总电压过高"
                n1591 = disable-structure shown="启用" {
                  disable-tunnel: [w4035 w4038] -> w4031
                  disable-tunnel: [w4034 w4038] -> w4030
                  disable-tunnel: w4028 -> [w4033 _]
                  frame Disabled {
                    n1592 = Unbundle By Name(w4033) -> ("总电压过高"=w4032:dbl)
                    n1593 = call "输入分辨率计算-EV05.vi"("1字节?"=FALSE, "数值"=w4032, "分辨率"=0.1) -> ("低字节"=w4035:dbl, "高字节1"=w4034:dbl)  [unwired: 2 in, 5 out]
                  }
                  frame Enabled {
                    w4038 = 255 ("高字节1")
                  }
                }
                n1594 = Build Array(w4030, w4031) -> (w4029:i32[])
              }
              frame 1 {
                # "总电压过低"
                n1595 = disable-structure shown="启用" {
                  disable-tunnel: [w4046 w4049] -> w4042
                  disable-tunnel: [w4045 w4049] -> w4041
                  disable-tunnel: w4039 -> [w4044 _]
                  frame Disabled {
                    n1596 = Unbundle By Name(w4044) -> ("总电压过低"=w4043:dbl)
                    n1597 = call "输入分辨率计算-EV05.vi"("1字节?"=FALSE, "数值"=w4043, "分辨率"=0.1) -> ("低字节"=w4046:dbl, "高字节1"=w4045:dbl)  [unwired: 2 in, 5 out]
                  }
                  frame Enabled {
                    w4049 = 255 ("高字节1")
                  }
                }
                n1598 = Build Array(w4041, w4042) -> (w4040:i32[])
              }
              frame 2 {
                # "温度过高"
                n1599 = disable-structure shown="启用" {
                  disable-tunnel: [w4056 255 ("高字节1")] -> w4052
                  disable-tunnel: w4050 -> [w4054 _]
                  frame Disabled {
                    n1600 = Unbundle By Name(w4054) -> ("温度过高"=w4053:dbl)
                    n1601 = call "输入分辨率计算-EV05.vi"("1字节?"=TRUE, "数值"=w4053, "偏移量"=-40.0, "分辨率"=1.0) -> ("高字节1"=w4056:dbl)  [unwired: 1 in, 6 out]
                  }
                  frame Enabled {
                  }
                }
                n1602 = Build Array(w4052) -> (w4051:i32[])
              }
              frame 3 {
                # "温度过低"
                n1603 = disable-structure shown="启用" {
                  disable-tunnel: [w4066 255 ("高字节1")] -> w4062
                  disable-tunnel: w4060 -> [w4064 _]
                  frame Disabled {
                    n1604 = Unbundle By Name(w4064) -> ("温度过低"=w4063:dbl)
                    n1605 = call "输入分辨率计算-EV05.vi"("1字节?"=TRUE, "数值"=w4063, "偏移量"=-40.0, "分辨率"=1.0) -> ("高字节1"=w4066:dbl)  [unwired: 1 in, 6 out]
                  }
                  frame Enabled {
                  }
                }
                n1606 = Build Array(w4062) -> (w4061:i32[])
              }
              frame 4 {
                # "整组温度不均衡"
                n1607 = disable-structure shown="启用" {
                  disable-tunnel: [w4075 255 ("高字节1")] -> w4072
                  disable-tunnel: w4070 -> [w4074 _]
                  frame Enabled {
                    n1608 = Unbundle By Name(w4074) -> ("整组温度不均衡"=w4073:dbl)
                    n1609 = call "输入分辨率计算-EV05.vi"("1字节?"=TRUE, "数值"=w4073, "分辨率"=1.0) -> ("高字节1"=w4075:dbl)  [unwired: 2 in, 6 out]
                  }
                  frame Disabled {
                  }
                }
                n1610 = Build Array(w4072) -> (w4071:dbl[])
              }
              frame 5 {
                # "单组电压不均衡"
                n1611 = disable-structure shown="启用" {
                  disable-tunnel: [w4087 w4090] -> w4082
                  disable-tunnel: [w4085 w4090] -> w4080
                  disable-tunnel: w4079 -> [w4084 _]
                  frame Disabled {
                    n1612 = Unbundle By Name(w4084) -> ("单组电压不均衡"=w4083:dbl)
                    n1613 = call "输入分辨率计算-EV05.vi"("1字节?"=FALSE, "数值"=w4083, "偏移量"=0.0, "分辨率"=0.001) -> ("低字节"=w4085:dbl, "高字节1"=w4087:dbl)  [unwired: 1 in, 5 out]
                  }
                  frame Enabled {
                    w4090 = 255 ("高字节1")
                  }
                }
                n1614 = Build Array(w4082, w4080) -> (w4081:i32[])
              }
              frame 6 {
                # "整组电压不均衡"
                n1615 = disable-structure shown="启用" {
                  disable-tunnel: [w4099 w4102] -> w4094
                  disable-tunnel: [w4097 w4102] -> w4092
                  disable-tunnel: w4091 -> [w4096 _]
                  frame Disabled {
                    n1616 = Unbundle By Name(w4096) -> ("整组电压不均衡"=w4095:dbl)
                    n1617 = call "输入分辨率计算-EV05.vi"("1字节?"=FALSE, "数值"=w4095, "偏移量"=0.0, "分辨率"=0.001) -> ("低字节"=w4097:dbl, "高字节1"=w4099:dbl)  [unwired: 1 in, 5 out]
                  }
                  frame Enabled {
                    w4102 = 255 ("高字节1")
                  }
                }
                n1618 = Build Array(w4094, w4092) -> (w4093:i32[])
              }
              frame 7 {
                # "单体电压过高"
                n1619 = disable-structure shown="启用" {
                  disable-tunnel: [w4111 w4114] -> w4106
                  disable-tunnel: [w4109 w4114] -> w4104
                  disable-tunnel: w4103 -> [w4108 _]
                  frame Disabled {
                    n1620 = Unbundle By Name(w4108) -> ("单体电压过高"=w4107:dbl)
                    n1621 = call "输入分辨率计算-EV05.vi"("1字节?"=FALSE, "数值"=w4107, "偏移量"=0.0, "分辨率"=0.001) -> ("低字节"=w4109:dbl, "高字节1"=w4111:dbl)  [unwired: 1 in, 5 out]
                  }
                  frame Enabled {
                    w4114 = 255 ("高字节1")
                  }
                }
                n1622 = Build Array(w4106, w4104) -> (w4105:i32[])
              }
              frame 8 {
                # "单体电压过低"
                n1623 = disable-structure shown="启用" {
                  disable-tunnel: [w4123 w4126] -> w4118
                  disable-tunnel: [w4121 w4126] -> w4116
                  disable-tunnel: w4115 -> [w4120 _]
                  frame Disabled {
                    n1624 = Unbundle By Name(w4120) -> ("单体电压过低"=w4119:dbl)
                    n1625 = call "输入分辨率计算-EV05.vi"("1字节?"=FALSE, "数值"=w4119, "偏移量"=0.0, "分辨率"=0.001) -> ("低字节"=w4121:dbl, "高字节1"=w4123:dbl)  [unwired: 1 in, 5 out]
                  }
                  frame Enabled {
                    w4126 = 255 ("高字节1")
                  }
                }
                n1626 = Build Array(w4118, w4116) -> (w4117:i32[])
              }
              frame 9 {
                # "充电电流过高"
                n1627 = disable-structure shown="启用" {
                  disable-tunnel: [w4135 w4138] -> w4130
                  disable-tunnel: [w4133 w4138] -> w4128
